vi "Query Trigger Connector Catalog.vi"(8 "error in (no error)":errorcluster, 11 "VISA resource name":refnum<visa-resource-name>) -> (0 "error out":errorcluster, 2 "Connectors":string, 3 "VISA resource name out":refnum<visa-resource-name>)   [LabVIEW 2015, in "Rohde&Schwarz CMXP Base.lvlib"]
doc: "Lists all trigger connectors of the primary instrument and of all instruments controlled by the primary instrument.\n\nIn a multi-box setup, a number <n> is returned for the styles NAME and FQName. The number <n> identifies the instrument. If this command returns an <n> = 0, 1, ... then add 1 to get the value for the suffix <n> in the other commands (1, 2, ...).\n\nFor a single-box setup, the number <n> is omitted in the returned strings and you can omit the suffix <n> in the other commands.\n\nAttribute:\nRSCMXPBASE_ATTR_TRIGGER_CONNECTOR_CATALOG\n\nRemote-control command:\nTRIGger:BASE:EXTernal:CATalog?"
uses:
  <instrlib>/Rohde&Schwarz CMXP Base/Rohde&Schwarz CMXP Base.lvlib
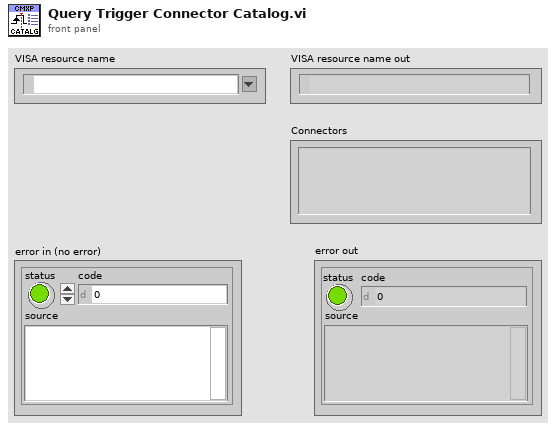
[diagram p1: front panel]
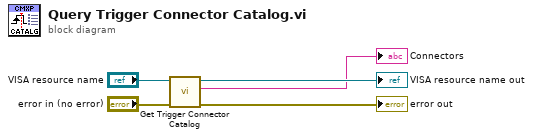
[diagram p0: block diagram]
diagram:
  n1 = call "Get Trigger Connector Catalog"("error in (no error)"="error in (no error)", "instrument handle"="VISA resource name") -> ("error out"=→"error out":errorcluster, "Trigger Connector Catalog"=→"Connectors":string, "instrument handle out"=→"VISA resource name out":refnum<visa-resource-name>)  [unwired: 7 in]
